vi "Initialize.vi"(7 "Channel Name":string="Setpoint.ch%d.SP", 8 "error in":errorcluster, 9 "Number of Channels":u32=1, 10 "Instance Name":string, 11 "Temperature Actual Value in":refnum<class "Temperature Actual Value.lvclass">) -> (0 "error out":errorcluster, 2 "Channel":T1[](array[typedef]), 3 "Temperature Actual Value out":refnum<class "Temperature Actual Value.lvclass">)   [LabVIEW 2023, in "Temperature Actual Value.lvclass"]
uses:
  Temperature Actual Value.lvclass
  Parents/Actual Value/Actual Value.lvclass
  Utilities/Channel.ctl
  Utilities/Utilities.lvlib
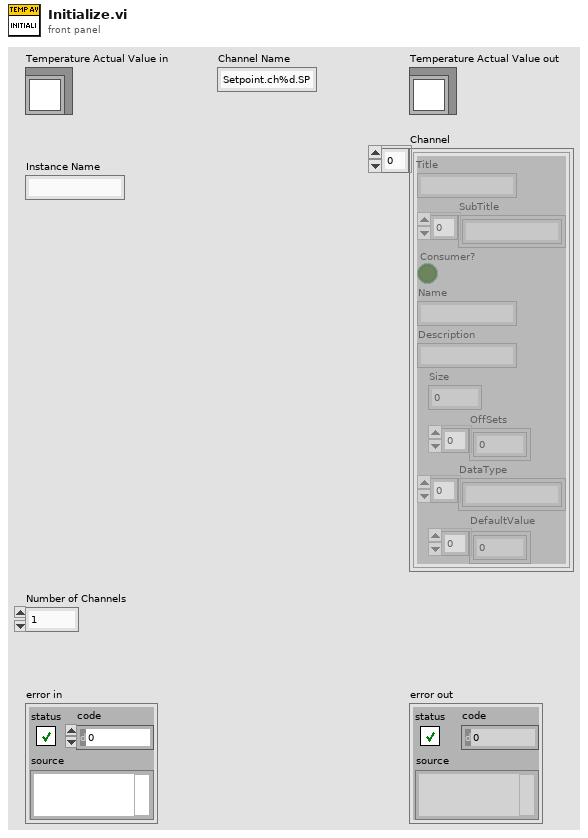
[diagram p1: front panel]
types:
  T1 = typedef "Utilities.lvlib/Channel.ctl" = cluster{"Title":string, "SubTitle":string[], "Consumer?":bool, "Name":string, "Description":string, "Size":i32, "OffSets":i32[], "DataType":string[], "DefaultValue":dbl[]}
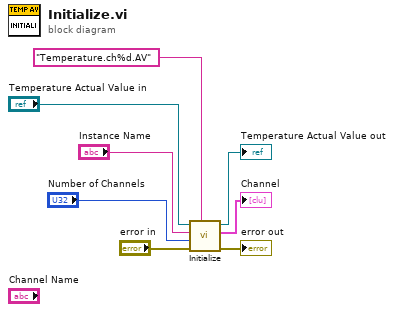
[diagram p0: block diagram]
diagram:
  n1 = call-parent "Initialize.vi"("Channel Name"="Temperature.ch%d.AV" ("ChannelName"), "error in"="error in", "Number of Channels"="Number of Channels", "Instance Name"="Instance Name", "Actual Value in"="Temperature Actual Value in") -> ("error out"=→"error out":errorcluster, "Channel"=→"Channel":T1[], "Actual Value out"=→"Temperature Actual Value out":refnum<class "Temperature Actual Value.lvclass">)  [unwired: 4 in]
